vi "Work.vi"(2 "ThreadIdIn":u32, 3 "Dll Path":path) -> (0 "CPUThreadAffinity":u32, 1 "UsedThreadId":u32)   [LabVIEW 2012]
panel:
  out "Counter":i32
  out "error out":errorcluster
  in  "stop":bool
  in  "error in (no error)":errorcluster
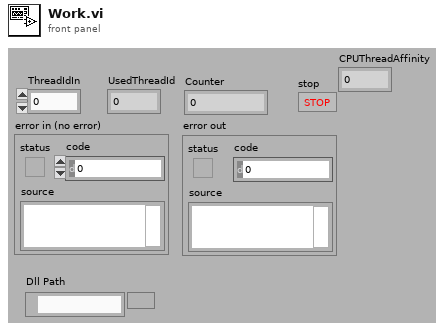
[diagram p1: front panel]
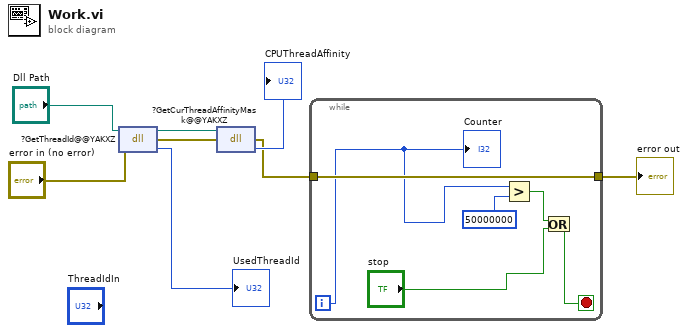
[diagram p0: block diagram]
diagram:
  n1 = dll-call lib="ThreadDll.dll" fn="?GetThreadId@@YAKXZ"(path in="Dll Path", error in="error in (no error)") -> (path out=w4:path, error out=w6:errorcluster, "return type"=→"UsedThreadId":u32)  [unwired: 1 in]
  n2 = dll-call lib="ThreadDll.dll" fn="?GetCurThreadAffinityMask@@YAKXZ"(path in=w4, error in=w6) -> (error out=w1:errorcluster, "return type"=→"CPUThreadAffinity":u32)  [unwired: 1 in, 1 out]
  n3 = while {
    tunnel: w1 -> [w14]
    tunnel: [w14] -> w3
    i -> [w12]
    stop <- w9 stop-if-true
    n4 = Greater?(x=w12, y=50000000) -> (0:w11:bool)
    n5 = Or(x=w11, y="stop") -> (x .or. y?=w9:bool)
    "Counter" <- w12
  }
  "error out" <- w3
